vi "Device Test.vi"(8 "error in (no error)":errorcluster) -> (0 "error out":errorcluster)   [LabVIEW 2011, in "Multimeter.lvclass"]
uses:
  Multimeter.lvclass
  Agilent 3458A/Agilent 3458A.lvclass
panel:
  in  "Integration Time":dbl
  in  "VISA resource name":refnum<visa-resource-name>
  in  "stop":bool
  out "Resistance":dbl
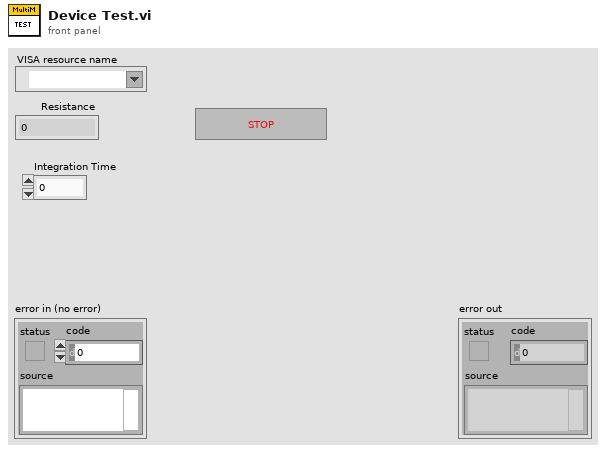
[diagram p1: front panel]
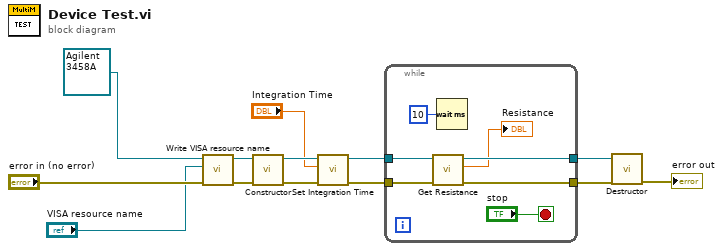
[diagram p0: block diagram]
diagram:
  n1 = call-dynamic "Write VISA resource name.vi"("error in (no error)"="error in (no error)", "VISA resource name"="VISA resource name", "Multimeter in"=refnum<class "Agilent 3458A.lvclass"> refnum ("Agilent 3458A.lvclass")) -> ("error out"=w8:errorcluster, "Multimeter out"=w7:refnum<class "Agilent 3458A.lvclass">)  [unwired: 7 in]
  n2 = call-dynamic "Constructor.vi"("error in (no error)"=w8, "Agilent 3458A in"=w7) -> ("error out"=w4:errorcluster, "Agilent 3458A out"=w5:refnum<class "Agilent 3458A.lvclass">)  [unwired: 7 in, 1 out]
  n3 = call-dynamic "Set Integration Time.vi"("error in (no error)"=w4, "Integration Time"="Integration Time", "Agilent 3458A in"=w5) -> ("error out"=w2:errorcluster, "Agilent 3458A out"=w3:refnum<class "Agilent 3458A.lvclass">)  [unwired: 7 in]
  n4 = while {
    tunnel: w2 -> [w20]
    tunnel: w3 -> [w19]
    tunnel: [w18] -> w12
    tunnel: [w17] -> w11
    stop <- "stop" stop-if-true
    n5 = call-dynamic "Get Resistance.vi"("error in (no error)"=w20, "Agilent 3458A in"=w19) -> ("error out"=w18:errorcluster, "Resistance"=→"Resistance":dbl, "Agilent 3458A out"=w17:refnum<class "Agilent 3458A.lvclass">)  [unwired: 7 in]
    n6 = Wait (ms)(milliseconds to wait=u32 10) -> ()  [unwired: 1 out]
  }
  n7 = call-dynamic "Destructor.vi"("error in (no error)"=w12, "Agilent 3458A in"=w11) -> ("error out"=→"error out":errorcluster)  [unwired: 8 in, 1 out]
